vi "Save Map.vi"(8 "error in (no error)":errorcluster, 11 "Map Model in":refnum<class "Map Model.lvclass">) -> (0 "error out":errorcluster, 3 "Map Model out":refnum<class "Map Model.lvclass">)   [LabVIEW 2020, in "Map Model.lvlib" / "Map Model.lvclass"]
uses:
  Map Model.lvclass
  Map Model.lvclass/Map Model.ctl
panel:
  # "NOTICE -- YOU MUST LEAVE THIS NOTICE IN PLACE.\n\nCopyright (c) 2017, LIANG LIU Shawn.Liu.cn@gmail.com\nAll rights reserved.\n\nRedistribution and use in source and binary forms, with or without modification, are permitted provided that the following conditions are met:\n-Redistributions of source code must retain the above copyright notice, this list of conditions and the following disclaimer.\n-Redistributions in binary form must reproduce the above copyright notice, this list of conditions and the following disclaimer in the documentation and/or other materials provided with the distribution.\n-Neither the name of the eLp nor the names of its contributors may be used to endorse or promote products derived from this software without specific prior written permission.\n\nTHIS SOFTWARE IS PROVIDED BY THE COPYRIGHT HOLDERS AND CONTRIBUTORS \"AS IS\" AND ANY EXPRESS OR IMPLIED WARRANTIES, INCLUDING, BUT NOT LIMITED TO, THE IMPLIED WARRANTIES OF MERCHANTABILITY AND FITNESS FOR A PARTICULAR PURPOSE ARE DISCLAIMED. IN NO EVENT SHALL THE COPYRIGHT HOLDER OR CONTRIBUTORS BE LIABLE FOR ANY DIRECT, INDIRECT, INCIDENTAL, SPECIAL, EXEMPLARY, OR CONSEQUENTIAL DAMAGES (INCLUDING, BUT NOT LIMITED TO, PROCUREMENT OF SUBSTITUTE GOODS OR SERVICES; LOSS OF USE, DATA, OR PROFITS; OR BUSINESS INTERRUPTION) HOWEVER CAUSED AND ON ANY THEORY OF LIABILITY, WHETHER IN CONTRACT, STRICT LIABILITY, OR TORT (INCLUDING NEGLIGENCE OR OTHERWISE) ARISING IN ANY WAY OUT OF THE USE OF THIS SOFTWARE, EVEN IF ADVISED OF THE POSSIBILITY OF SUCH DAMAGE."
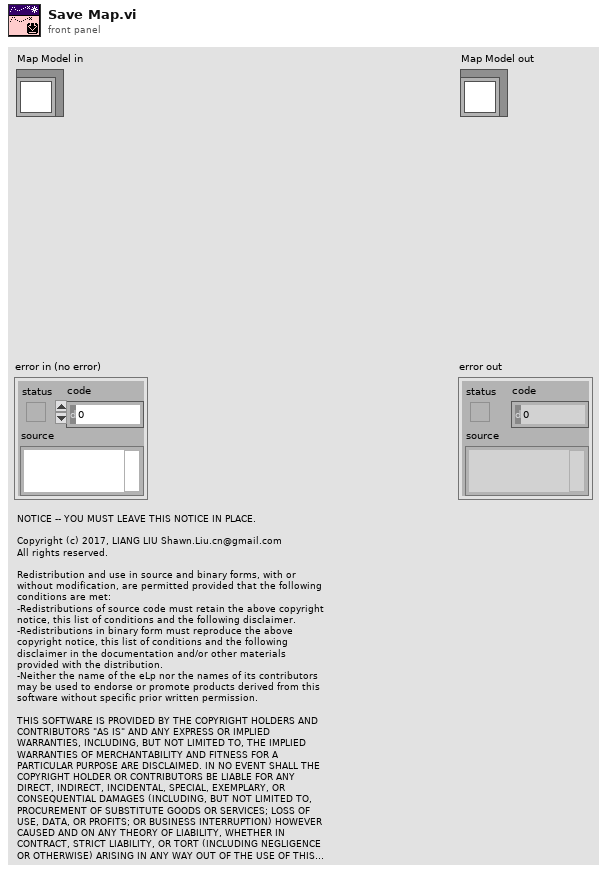
[diagram p1: front panel]
types:
  T1 = enum16{"open", "replace", "create", "open or create", "replace or create", "replace or create with confirmation"}
  T2 = cluster{"left":i16, "top":i16, "right":i16, "bottom":i16}
  T3 = typedef "imagedata.ctl" = cluster{"image type":i32, "image depth":i32, "image":u8[], "mask":u8[], "colors":u32[], "Rectangle":cluster{"left":i16, "top":i16, "right":i16, "bottom":i16}}
  T4 = cluster{"Occupied Color":cluster{"Value":u8, "Color":u32}, "Free Color":cluster{"Value":u8, "Color":u32}, "Unknown Color":cluster{"Value":u8, "Color":u32}}
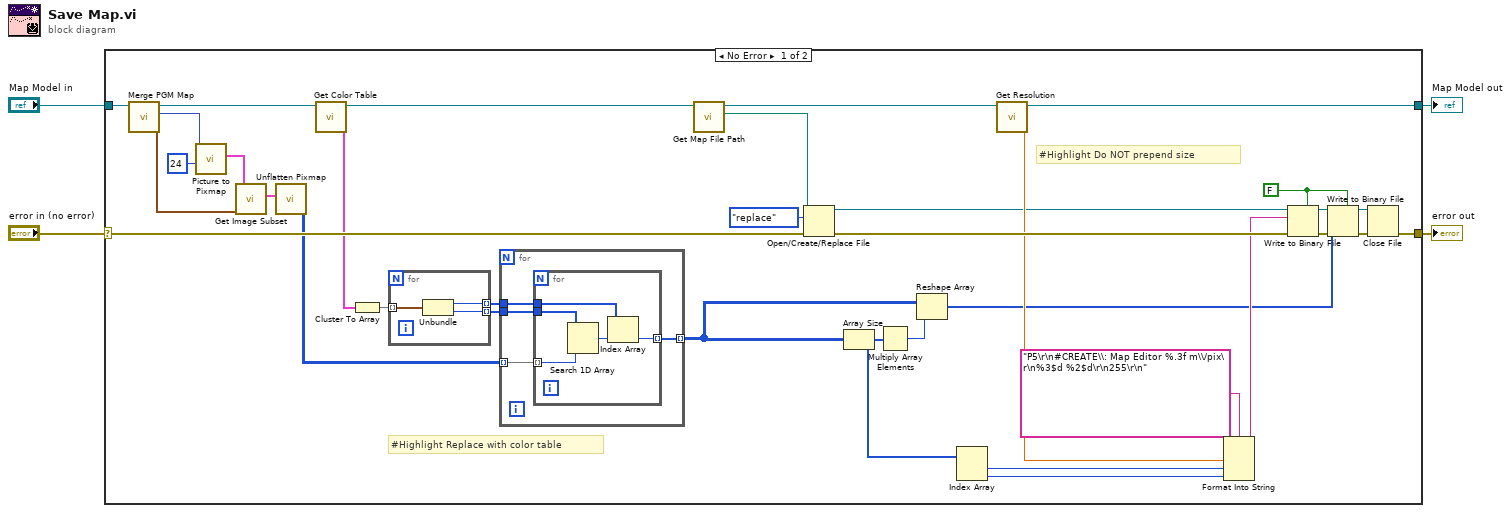
[diagram p0: block diagram]
diagram:
  n1 = case shown="No Error" "error in (no error)" {
    selector: "error in (no error)" -> [w39 w53]
    tunnel: [w38 w52] -> w3
    tunnel: [w37 w53] -> w2
    tunnel: "Map Model in" -> [w36 w52]
    frame No Error {
      w9 = FALSE ("prepend array or string size? (T)")
      # "#Highlight Do NOT prepend size"
      # "#Highlight Replace with color table"
      n2 = call "Merge PGM Map.vi"("Map Model in"=w36) -> ("Map Rectangle"=w6:T2, "Map"=w8:picture, "Map Model out"=w18:refnum<class "Map Model.lvclass">)  [unwired: 7 in, 1 out]
      n3 = call <vilib>:"Picture to Pixmap.vi"("depth"=24, "picture"=w8) -> ("image data"=w7:T3)  [unwired: 8 in, 1 out]
      n4 = call <vilib>:"Get Image Subset.vi"("subset rect"=w6, "image data"=w7) -> ("image subset"=w10:T3)  [unwired: 4 in, 1 out]
      n5 = call <vilib>:"Unflatten Pixmap.vi"("image data"=w10) -> ("24-bit pixmap"=w5:u32[][])  [unwired: 4 in, 6 out]
      n6 = call "Get Color Table.vi"("Map Model in"=w18) -> ("Color Table"=w15:T4, "Map Model out"=w16:refnum<class "Map Model.lvclass">)  [unwired: 9 in]
      n7 = Cluster To Array(cluster=w15) -> (array=w14:cluster{"Value":u8, "Color":u32}[])
      n8 = for {
        tunnel: w14 -> [w42] mode=indexing
        tunnel: [w41] -> w12 mode=indexing
        tunnel: [w40] -> w13 mode=indexing
        n9 = Unbundle(w42) -> ("Value"=w41:u8, "Color"=w40:u32)
      }
      n10 = for {
        tunnel: w5 -> [w46] mode=indexing
        tunnel: [w45] -> w11 mode=indexing
        tunnel: w13 -> [w44]
        tunnel: w12 -> [w43]
        n11 = for {
          tunnel: w46 -> [w47] mode=indexing
          tunnel: [w49] -> w45 mode=indexing
          tunnel: w44 -> [w48]
          tunnel: w43 -> [w51]
          n12 = Search 1D Array(1D array=w48, element=w47) -> (index of element=w50:i32)  [unwired: 1 in]
          n13 = Index Array(array=w51, index=w50) -> (element=w49:u8)
        }
      }
      n14 = call "Get Map File Path.vi"("Map Model in"=w16) -> ("Map File Path"=w31:path, "Map Model out"=w35:refnum<class "Map Model.lvclass">)  [unwired: 9 in]
      n15 = Open/Create/Replace File(file path (use dialog)=w31, error in=w39, operation (0:open)=T1."replace") -> (refnum out=w24:refnum<file>, error out=w33:errorcluster)  [unwired: 3 in, 1 out]
      n16 = Array Size(array=w11) -> (size(s)=w28:i32[])
      n17 = Multiply Array Elements(1:w28) -> (0:w34:i32)
      n18 = Reshape Array(w11, w34) -> (w20:u8[])
      n19 = Index Array(array=w28) -> (element #1=w27:i32, element #2=w26:i32)  [unwired: 2 in]
      n20 = call "Get Resolution.vi"("Map Model in"=w35) -> ("Resolution"=w25:dbl, "Map Model out"=w38:refnum<class "Map Model.lvclass">)  [unwired: 9 in]
      n21 = Format Into String(format string="P5\r\n#CREATE\\: Map Editor %.3f m\\/pix\r\n%3$d %2$d\r\n255\r\n", w25, w27, w26) -> (resulting string=w23:string)  [unwired: 2 in, 1 out]
      n22 = Write to Binary File(file (use dialog)=w24, data=w23, error in=w33, 5:w9) -> (refnum out=w21:refnum<file>, error out=w30:errorcluster)  [unwired: 2 in, 1 out]
      n23 = Write to Binary File(file (use dialog)=w21, data=w20, error in=w30, 5:w9) -> (refnum out=w19:refnum<file>, error out=w22:errorcluster)  [unwired: 2 in, 1 out]
      n24 = Close File(refnum=w19, error in=w22) -> (error out=w37:errorcluster)  [unwired: 1 out]
    }
    frame Error {
    }
  }
  "error out" <- w2
  "Map Model out" <- w3
